vi "Write Elevation.vi"(8 "error in (no error)":errorcluster, 10 "elevation":dbl[unit] min=-0.08726646259971647 max=1.6580627893946132, 11 "MccAzElMove in":refnum<class "MccAzElMove.lvclass">) -> (0 "error out":errorcluster, 3 "MccAzElMove out":refnum<class "MccAzElMove.lvclass">)   [LabVIEW 2014, in "TCSDataDefinitions.lvlib" / "TCSMountControlCommand.lvlib" / "CommandsForAzElAxes.lvlib" / "MccAzElMove.lvclass"]
uses:
  MccAzElMove.lvclass
  MccAzElMove.lvclass/MccAzElMove.ctl
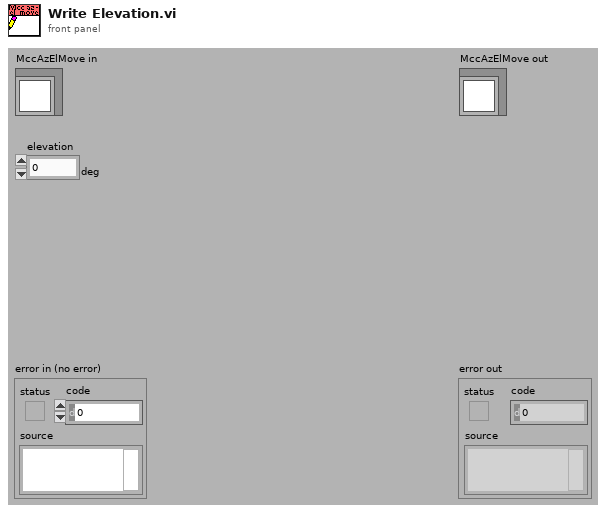
[diagram p1: front panel]
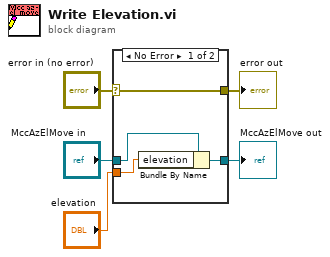
[diagram p0: block diagram]
diagram:
  n1 = case shown="No Error" "error in (no error)" {
    selector: "error in (no error)" -> [w9 w10]
    tunnel: [w9 w10] -> w4
    tunnel: [w7 w11] -> w2
    tunnel: "MccAzElMove in" -> [w8 w11]
    tunnel: "elevation" -> [w6 _]
    frame No Error {
      n2 = Bundle By Name(cluster=w8, "elevation"=w6) -> (w7:refnum<class "MccAzElMove.lvclass">)
    }
    frame Error {
    }
  }
  "error out" <- w4
  "MccAzElMove out" <- w2
